vi "Get Image ROI Contour.vi"(7 "Image Model":T1, 8 "Error In":errorcluster, 10 "ROI Descriptor":T2 {"Contours"."Type" items=["No Selection", "Point", "Line", "Rectangle", "Oval", "Polygon", "Freehand Region", "Annulus", "Unused2", "Unused3", "Broken Line", "Freehand Line", "Rotated Rectangle"]}, 11 "ROI Mask":T1) -> (0 "Error Out":errorcluster, 2 "ROI Contour Descriptor":T2 {"Contours"."Type" items=["No Selection", "Point", "Line", "Rectangle", "Oval", "Polygon", "Freehand Region", "Annulus", "Unused2", "Unused3", "Broken Line", "Freehand Line", "Rotated Rectangle"]})   [LabVIEW 2021, in "Image.lvlib"]
uses:
  Image.lvlib
  <vilib>/vision/Image Controls.llb/IMAQ Image.ctl
  <vilib>/vision/NI_Vision_Development_Module.lvlib
  Strings/Strings.lvlib
  Error/Error.lvlib
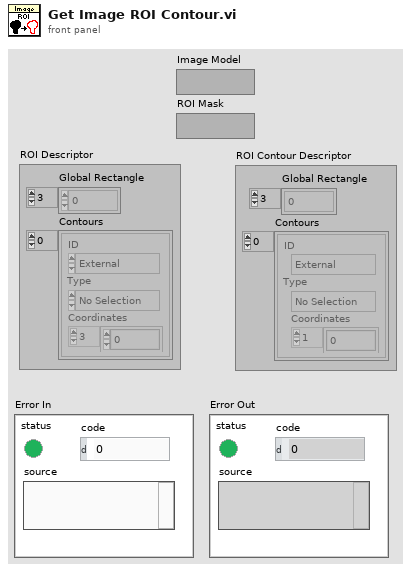
[diagram p1: front panel]
types:
  T1 = typedef "IMAQ Image.ctl" = refnum<image>
  T2 = typedef "ROI Descriptor" = cluster{"Global Rectangle":i32[], "Contours":cluster{"ID":enum32{"External", "Internal"}, "Type":u32, "Coordinates":i32[]}[]}
  T3 = cluster{"ID":enum32{"External", "Internal"}, "Type":u32, "Coordinates":i32[]}[]
  T4 = cluster{"ID":enum32{"External", "Internal"}, "Type":u32, "Coordinates":i32[]}
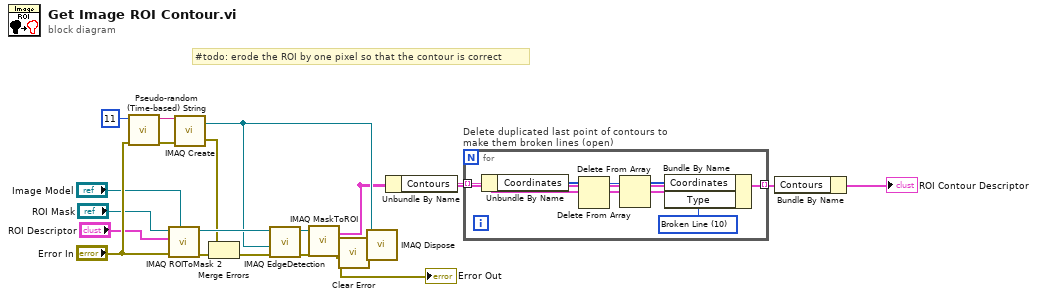
[diagram p0: block diagram]
diagram:
  # "#todo: erode the ROI by one pixel so that the contour is correct"
  n1 = call "Pseudo-random (Time-based) String.vi"("Error In"="Error In", "Length (10)"=u32 11) -> ("Error Out"=w18:errorcluster, "result string"=w15:string)  [unwired: 8 in]
  n2 = call "IMAQ ROIToMask 2"("Image Model"="Image Model", "error in (no error)"="Error In", "ROI Descriptor"="ROI Descriptor", "Image"="ROI Mask") -> ("error out"=w20:errorcluster, "Image Out"=w19:T1)  [unwired: 5 in, 1 out]
  n3 = call "IMAQ Create"("Image Name"=w15, "error in (no error)"=w18) -> ("New Image"=w7:T1, "error out"=w8:errorcluster)  [unwired: 3 in]
  n4 = Merge Errors(w8, w20) -> (w14:errorcluster)
  n5 = call "IMAQ EdgeDetection"("error in (no error)"=w14, "Image Dst"=w7, "Image Src"=w19) -> ("error out"=w12:errorcluster, "Image Dst Out"=w13:T1)  [unwired: 7 in]
  n6 = call "IMAQ MaskToROI"("Image"=w13, "error in (no error)"=w12) -> ("ROI Descriptor"=w6:T2, "error out"=w1:errorcluster)  [unwired: 5 in, 1 out]
  "Error Out" <- w1
  n7 = call "Clear Error.vi"("Error In"=w1) -> ("no Error Out"=w2:errorcluster)  [unwired: 8 in]
  n8 = call "IMAQ Dispose"("Image"=w7, "error in (no error)"=w2) -> ()  [unwired: 4 in, 1 out]
  n9 = Unbundle By Name(w6) -> ("Contours"=w4:T3)
  n10 = for "Delete duplicated last point of contours to make them broken lines (open)" {
    tunnel: w4 -> [w26] mode=indexing
    tunnel: [w24] -> w3 mode=indexing
    w25 = u32 10 items=["No Selection", "Point", "Line", "Rectangle", "Oval", "Polygon", "Freehand Region", "Annulus", "Unused2", "Unused3", "Broken Line", "Freehand Line", "Rotated Rectangle"] ("Type")
    n11 = Unbundle By Name(w26) -> ("Coordinates"=w23:i32[])
    n12 = Delete From Array(array=w23) -> (array with subset deleted=w22:i32[])  [unwired: 2 in, 1 out]
    n13 = Delete From Array(array=w22) -> (array with subset deleted=w21:i32[])  [unwired: 2 in, 1 out]
    n14 = Bundle By Name(cluster=w26, "Coordinates"=w21, "Type"=w25) -> (w24:T4)
  }
  n15 = Bundle By Name(cluster=w6, "Contours"=w3) -> (→"ROI Contour Descriptor":T2)
